vi "Perform Action.vi"(8 "error in (no error)":errorcluster, 10 "Input":variant, 11 "Thermometer DAQmx Base CFG in":refnum<class "Thermometer DAQmx Base CFG.lvclass">) -> (0 "error out":errorcluster, 2 "Output":variant, 3 "Thermometer DAQmx Base CFG out":refnum<class "Thermometer DAQmx Base CFG.lvclass">)   [LabVIEW 2023, in "Thermometer DAQmx Base CFG.lvclass"]
uses:
  Thermometer DAQmx Base CFG.lvclass
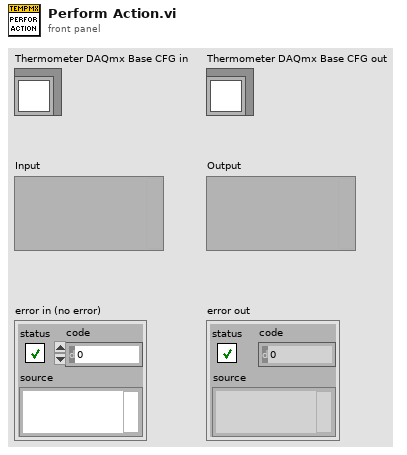
[diagram p1: front panel]
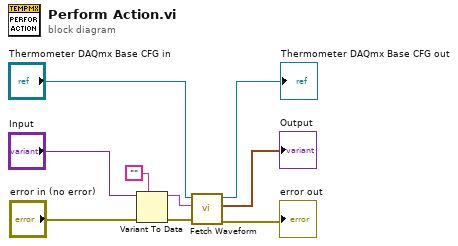
[diagram p0: block diagram]
diagram:
  n1 = Variant To Data(error in="error in (no error)", type="", Variant="Input") -> (data=w6:string, error out=w8:errorcluster)
  n2 = call-dynamic "Fetch Waveform.vi"("error in (no error)"=w8, "Channel"=w6, "Thermometer DAQmx Base CFG in"="Thermometer DAQmx Base CFG in") -> ("error out"=→"error out":errorcluster, "Waveform"=→"Output":waveform(dbl), "Thermometer DAQmx Base CFG out"=→"Thermometer DAQmx Base CFG out":refnum<class "Thermometer DAQmx Base CFG.lvclass">)  [unwired: 6 in]
